vi "GetNames.vi"(11 "Proccess in":refnum<class "Proccess.lvclass">) -> (2 "Tags":T1)   [LabVIEW 2019, in "Proccess.lvclass"]
uses:
  Proccess.lvclass
  TAGs.ctl
  Proccess.lvclass/Proccess.ctl
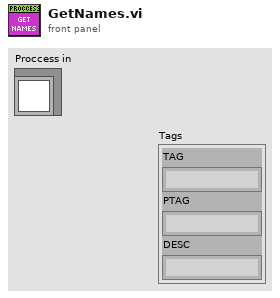
[diagram p1: front panel]
types:
  T1 = typedef "Proccess.lvclass/TAGs.ctl" = cluster{"TAG":string, "PTAG":string, "DESC":string}
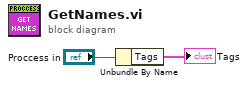
[diagram p0: block diagram]
diagram:
  n1 = Unbundle By Name("Proccess in") -> ("Tags"=→"Tags":T1)
